vi "GetTileNumberTool.vi"() -> ()   [LabVIEW 2019, in "Initializers.lvlib"]
uses:
  Initializers.lvlib
  <vilib>/Utility/miscctls.llb/LVPositionTypeDef.ctl
panel:
  out "Tilecode":u32=134217750
  in  "Flip":enum16{"None", "LeftRight", "UpDown", "Both"}(ring)
  in  "replace_color 2":fxp<+,3,3>
  in  "color_to_replace 2":fxp<+,3,3>
  out "TileNumber":u32=134217750
  in  "replace_color":fxp<+,3,3>
  in  "color_to_replace":fxp<+,3,3>=2.0
  out "element":picture
  in  "Rotation":enum16{"None", "Right", "Down", "Left"}(ring)
  in  "ReloadFile":bool
  out "Array 2":picture[][](array[picture])=[[bytes[830], bytes[830], bytes[830], bytes[830], bytes[830], bytes[830], bytes[830], bytes[830], bytes[830], bytes[830], bytes[830], bytes[830], bytes[830], bytes[830], bytes[830], bytes[830], bytes[798], bytes[798], bytes[798], bytes[798], bytes[798], bytes[798], bytes[798], bytes[798], bytes[798], bytes[798], bytes[798], bytes[798], bytes[798], bytes[798], bytes[798], bytes[798], bytes[798], bytes[798], bytes[798], bytes[798], bytes[798], bytes[798], bytes[798], bytes[798], bytes[798], bytes[798], bytes[798], bytes[798], bytes[798], bytes[798], bytes[798], bytes[798], bytes[798], bytes[798], bytes[798], bytes[798], bytes[798], bytes[798], bytes[798], bytes[798], bytes[798], bytes[798], bytes[798], bytes[798], bytes[798], bytes[798], bytes[798], bytes[798]], [bytes[830], bytes[830], bytes[830], bytes[830], bytes[830], bytes[830], bytes[830], bytes[830], bytes[830], bytes[830], bytes[830], bytes[830], bytes[830], bytes[830], bytes[830], bytes[830], bytes[798], bytes[798], bytes[798], bytes[798], bytes[798], bytes[798], bytes[798], bytes[798], bytes[798], bytes[798], bytes[798], bytes[798], bytes[798], bytes[798], bytes[798], bytes[798], bytes[798], bytes[798], bytes[798], bytes[798], bytes[798], bytes[798], bytes[798], bytes[798], bytes[798], bytes[798], bytes[798], bytes[798], bytes[798], bytes[798], bytes[798], bytes[798], bytes[798], bytes[798], bytes[798], bytes[798], bytes[798], bytes[798], bytes[798], bytes[798], bytes[798], bytes[798], bytes[798], bytes[798], bytes[798], bytes[798], bytes[798], bytes[798]], [bytes[830], bytes[830], bytes[830], bytes[830], bytes[830], bytes[830], bytes[830], bytes[830], bytes[830], bytes[830], bytes[830], bytes[830], bytes[830], bytes[830], bytes[830], bytes[830], bytes[798], bytes[798], bytes[798], bytes[798], bytes[798], bytes[798], bytes[798], bytes[798], bytes[798], bytes[798], bytes[798], bytes[798], bytes[798], bytes[798], bytes[798], bytes[798], bytes[798], bytes[798], bytes[798], bytes[798], bytes[798], bytes[798], bytes[798], bytes[798], bytes[798], bytes[798], bytes[798], bytes[798], bytes[798], bytes[798], bytes[798], bytes[798], bytes[798], bytes[798], bytes[798], bytes[798], bytes[798], bytes[798], bytes[798], bytes[798], bytes[798], bytes[798], bytes[798], bytes[798], bytes[798], bytes[798], bytes[798], bytes[798]], [bytes[830], bytes[830], bytes[830], bytes[830], bytes[830], bytes[830], bytes[830], bytes[830], bytes[830], bytes[830], bytes[830], bytes[830], bytes[830], bytes[830], bytes[830], bytes[830], bytes[798], bytes[798], bytes[798], bytes[798], bytes[798], bytes[798], bytes[798], bytes[798], bytes[798], bytes[798], bytes[798], bytes[798], bytes[798], bytes[798], bytes[798], bytes[798], bytes[798], bytes[798], bytes[798], bytes[798], bytes[798], bytes[798], bytes[798], bytes[798], bytes[798], bytes[798], bytes[798], bytes[798], bytes[798], bytes[798], bytes[798], bytes[798], bytes[798], bytes[798], bytes[798], bytes[798], bytes[798], bytes[798], bytes[798], bytes[798], bytes[798], bytes[798], bytes[798], bytes[798], bytes[798], bytes[798], bytes[798], bytes[798]], [bytes[830], bytes[830], bytes[830], bytes[830], bytes[830], bytes[830], bytes[830], bytes[830], bytes[830], bytes[830], bytes[830], bytes[830], bytes[830], bytes[830], bytes[830], bytes[830], bytes[798], bytes[798], bytes[798], bytes[798], bytes[798], bytes[798], bytes[798], bytes[798], bytes[798], bytes[798], bytes[798], bytes[798], bytes[798], bytes[798], bytes[798], bytes[798], bytes[798], bytes[798], bytes[798], bytes[798], bytes[798], bytes[798], bytes[798], bytes[798], bytes[798], bytes[798], bytes[798], bytes[798], bytes[798], bytes[798], bytes[798], bytes[798], bytes[798], bytes[798], bytes[798], bytes[798], bytes[798], bytes[798], bytes[798], bytes[798], bytes[798], bytes[798], bytes[798], bytes[798], bytes[798], bytes[798], bytes[798], bytes[798]], [bytes[830], bytes[830], bytes[830], bytes[830], bytes[830], bytes[830], bytes[830], bytes[830], bytes[830], bytes[830], bytes[830], bytes[830], bytes[830], bytes[830], bytes[830], bytes[830], bytes[798], bytes[798], bytes[798], bytes[798], bytes[798], bytes[798], bytes[798], bytes[798], bytes[798], bytes[798], bytes[798], bytes[798], bytes[798], bytes[798], bytes[798], bytes[798], bytes[798], bytes[798], bytes[798], bytes[798], bytes[798], bytes[798], bytes[798], bytes[798], bytes[798], bytes[798], bytes[798], bytes[798], bytes[798], bytes[798], bytes[798], bytes[798], bytes[798], bytes[798], bytes[798], bytes[798], bytes[798], bytes[798], bytes[798], bytes[798], bytes[798], bytes[798], bytes[798], bytes[798], bytes[798], bytes[798], bytes[798], bytes[798]], [bytes[830], bytes[830], bytes[830], bytes[830], bytes[830], bytes[830], bytes[830], bytes[830], bytes[830], bytes[830], bytes[830], bytes[830], bytes[830], bytes[830], bytes[830], bytes[830], bytes[798], bytes[798], bytes[798], bytes[798], bytes[798], bytes[798], bytes[798], bytes[798], bytes[798], bytes[798], bytes[798], bytes[798], bytes[798], bytes[798], bytes[798], bytes[798], bytes[798], bytes[798], bytes[798], bytes[798], bytes[798], bytes[798], bytes[798], bytes[798], bytes[798], bytes[798], bytes[798], bytes[798], bytes[798], bytes[798], bytes[798], bytes[798], bytes[798], bytes[798], bytes[798], bytes[798], bytes[798], bytes[798], bytes[798], bytes[798], bytes[798], bytes[798], bytes[798], bytes[798], bytes[798], bytes[798], bytes[798], bytes[798]], [bytes[830], bytes[830], bytes[830], bytes[830], bytes[830], bytes[830], bytes[830], bytes[830], bytes[830], bytes[830], bytes[830], bytes[830], bytes[830], bytes[830], bytes[830], bytes[830], bytes[798], bytes[798], bytes[798], bytes[798], bytes[798], bytes[798], bytes[798], bytes[798], bytes[798], bytes[798], bytes[798], bytes[798], bytes[798], bytes[798], bytes[798], bytes[798], bytes[798], bytes[798], bytes[798], bytes[798], bytes[798], bytes[798], bytes[798], bytes[798], bytes[798], bytes[798], bytes[798], bytes[798], bytes[798], bytes[798], bytes[798], bytes[798], bytes[798], bytes[798], bytes[798], bytes[798], bytes[798], bytes[798], bytes[798], bytes[798], bytes[798], bytes[798], bytes[798], bytes[798], bytes[798], bytes[798], bytes[798], bytes[798]], [bytes[830], bytes[830], bytes[830], bytes[830], bytes[830], bytes[830], bytes[830], bytes[830], bytes[830], bytes[830], bytes[830], bytes[830], bytes[830], bytes[830], bytes[830], bytes[830], bytes[798], bytes[798], bytes[798], bytes[798], bytes[798], bytes[798], bytes[798], bytes[798], bytes[798], bytes[798], bytes[798], bytes[798], bytes[798], bytes[798], bytes[798], bytes[798], bytes[798], bytes[798], bytes[798], bytes[798], bytes[798], bytes[798], bytes[798], bytes[798], bytes[798], bytes[798], bytes[798], bytes[798], bytes[798], bytes[798], bytes[798], bytes[798], bytes[798], bytes[798], bytes[798], bytes[798], bytes[798], bytes[798], bytes[798], bytes[798], bytes[798], bytes[798], bytes[798], bytes[798], bytes[798], bytes[798], bytes[798], bytes[798]], [bytes[830], bytes[830], bytes[830], bytes[830], bytes[830], bytes[830], bytes[830], bytes[830], bytes[830], bytes[830], bytes[830], bytes[830], bytes[830], bytes[830], bytes[830], bytes[830], bytes[798], bytes[798], bytes[798], bytes[798], bytes[798], bytes[798], bytes[798], bytes[798], bytes[798], bytes[798], bytes[798], bytes[798], bytes[798], bytes[798], bytes[798], bytes[798], bytes[798], bytes[798], bytes[798], bytes[798], bytes[798], bytes[798], bytes[798], bytes[798], bytes[798], bytes[798], bytes[798], bytes[798], bytes[798], bytes[798], bytes[798], bytes[798], bytes[798], bytes[798], bytes[798], bytes[798], bytes[798], bytes[798], bytes[798], bytes[798], bytes[798], bytes[798], bytes[798], bytes[798], bytes[798], bytes[798], bytes[798], bytes[798]], [bytes[830], bytes[830], bytes[830], bytes[830], bytes[830], bytes[830], bytes[830], bytes[830], bytes[830], bytes[830], bytes[830], bytes[830], bytes[830], bytes[830], bytes[830], bytes[830], bytes[798], bytes[798], bytes[798], bytes[798], bytes[798], bytes[798], bytes[798], bytes[798], bytes[798], bytes[798], bytes[798], bytes[798], bytes[798], bytes[798], bytes[798], bytes[798], bytes[798], bytes[798], bytes[798], bytes[798], bytes[798], bytes[798], bytes[798], bytes[798], bytes[798], bytes[798], bytes[798], bytes[798], bytes[798], bytes[798], bytes[798], bytes[798], bytes[798], bytes[798], bytes[798], bytes[798], bytes[798], bytes[798], bytes[798], bytes[798], bytes[798], bytes[798], bytes[798], bytes[798], bytes[798], bytes[798], bytes[798], bytes[798]], [bytes[830], bytes[830], bytes[830], bytes[830], bytes[830], bytes[830], bytes[830], bytes[830], bytes[830], bytes[830], bytes[830], bytes[830], bytes[830], bytes[830], bytes[830], bytes[830], bytes[798], bytes[798], bytes[798], bytes[798], bytes[798], bytes[798], bytes[798], bytes[798], bytes[798], bytes[798], bytes[798], bytes[798], bytes[798], bytes[798], bytes[798], bytes[798], bytes[798], bytes[798], bytes[798], bytes[798], bytes[798], bytes[798], bytes[798], bytes[798], bytes[798], bytes[798], bytes[798], bytes[798], bytes[798], bytes[798], bytes[798], bytes[798], bytes[798], bytes[798], bytes[798], bytes[798], bytes[798], bytes[798], bytes[798], bytes[798], bytes[798], bytes[798], bytes[798], bytes[798], bytes[798], bytes[798], bytes[798], bytes[798]], [bytes[830], bytes[830], bytes[830], bytes[830], bytes[830], bytes[830], bytes[830], bytes[830], bytes[830], bytes[830], bytes[830], bytes[830], bytes[830], bytes[830], bytes[830], bytes[830], bytes[798], bytes[798], bytes[798], bytes[798], bytes[798], bytes[798], bytes[798], bytes[798], bytes[798], bytes[798], bytes[798], bytes[798], bytes[798], bytes[798], bytes[798], bytes[798], bytes[798], bytes[798], bytes[798], bytes[798], bytes[798], bytes[798], bytes[798], bytes[798], bytes[798], bytes[798], bytes[798], bytes[798], bytes[798], bytes[798], bytes[798], bytes[798], bytes[798], bytes[798], bytes[798], bytes[798], bytes[798], bytes[798], bytes[798], bytes[798], bytes[798], bytes[798], bytes[798], bytes[798], bytes[798], bytes[798], bytes[798], bytes[798]], [bytes[830], bytes[830], bytes[830], bytes[830], bytes[830], bytes[830], bytes[830], bytes[830], bytes[830], bytes[830], bytes[830], bytes[830], bytes[830], bytes[830], bytes[830], bytes[830], bytes[798], bytes[798], bytes[798], bytes[798], bytes[798], bytes[798], bytes[798], bytes[798], bytes[798], bytes[798], bytes[798], bytes[798], bytes[798], bytes[798], bytes[798], bytes[798], bytes[798], bytes[798], bytes[798], bytes[798], bytes[798], bytes[798], bytes[798], bytes[798], bytes[798], bytes[798], bytes[798], bytes[798], bytes[798], bytes[798], bytes[798], bytes[798], bytes[798], bytes[798], bytes[798], bytes[798], bytes[798], bytes[798], bytes[798], bytes[798], bytes[798], bytes[798], bytes[798], bytes[798], bytes[798], bytes[798], bytes[798], bytes[798]], [bytes[830], bytes[830], bytes[830], bytes[830], bytes[830], bytes[830], bytes[830], bytes[830], bytes[830], bytes[830], bytes[830], bytes[830], bytes[830], bytes[830], bytes[830], bytes[830], bytes[798], bytes[798], bytes[798], bytes[798], bytes[798], bytes[798], bytes[798], bytes[798], bytes[798], bytes[798], bytes[798], bytes[798], bytes[798], bytes[798], bytes[798], bytes[798], bytes[798], bytes[798], bytes[798], bytes[798], bytes[798], bytes[798], bytes[798], bytes[798], bytes[798], bytes[798], bytes[798], bytes[798], bytes[798], bytes[798], bytes[798], bytes[798], bytes[798], bytes[798], bytes[798], bytes[798], bytes[798], bytes[798], bytes[798], bytes[798], bytes[798], bytes[798], bytes[798], bytes[798], bytes[798], bytes[798], bytes[798], bytes[798]], [bytes[830], bytes[830], bytes[830], bytes[830], bytes[830], bytes[830], bytes[830], bytes[830], bytes[830], bytes[830], bytes[830], bytes[830], bytes[830], bytes[830], bytes[830], bytes[830], bytes[798], bytes[798], bytes[798], bytes[798], bytes[798], bytes[798], bytes[798], bytes[798], bytes[798], bytes[798], bytes[798], bytes[798], bytes[798], bytes[798], bytes[798], bytes[798], bytes[798], bytes[798], bytes[798], bytes[798], bytes[798], bytes[798], bytes[798], bytes[798], bytes[798], bytes[798], bytes[798], bytes[798], bytes[798], bytes[798], bytes[798], bytes[798], bytes[798], bytes[798], bytes[798], bytes[798], bytes[798], bytes[798], bytes[798], bytes[798], bytes[798], bytes[798], bytes[798], bytes[798], bytes[798], bytes[798], bytes[798], bytes[798]]]
  in  "path to PNG file":path=path "C:/Users/FreshBob/Dropbox/VIs/myRIO_GameConsole/Data/Tilesets/UnifiedTileset.png"
  in  "stop":bool
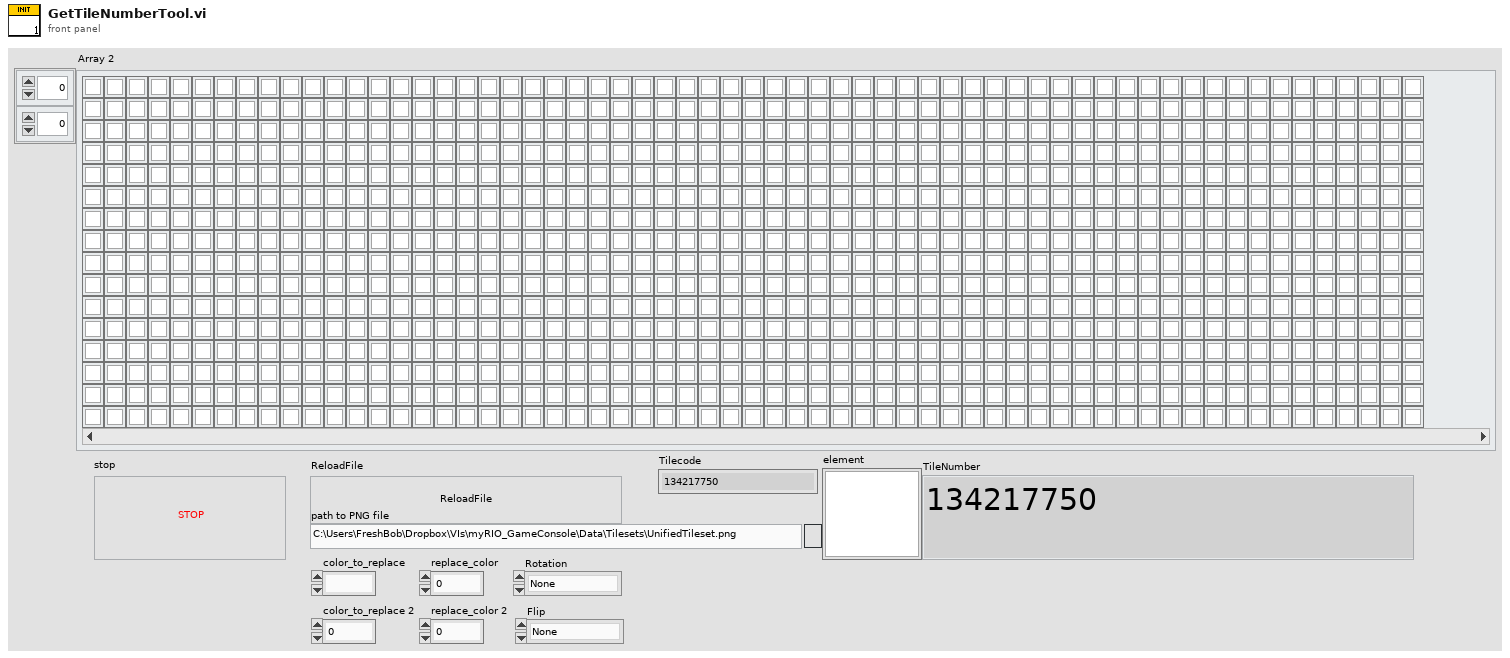
[diagram p1: front panel]
types:
  T1 = typedef "LVPositionTypeDef.ctl" = cluster{"Left":i32, "Top":i32}
  T2 = cluster{"left":i16, "top":i16, "right":i16, "bottom":i16}
  T3 = typedef "LVPoint32TypeDef.ctl" = cluster{"Horizontal":i32, "Vertical":i32}
  T4 = typedef "LVBoundsTypeDef.ctl" = cluster{"Width":u32, "Height":u32}
  T5 = typedef "imagedata.ctl" = cluster{"image type":i32, "image depth":i32, "image":u8[], "mask":u8[], "colors":u32[], "Rectangle":cluster{"left":i16, "top":i16, "right":i16, "bottom":i16}}
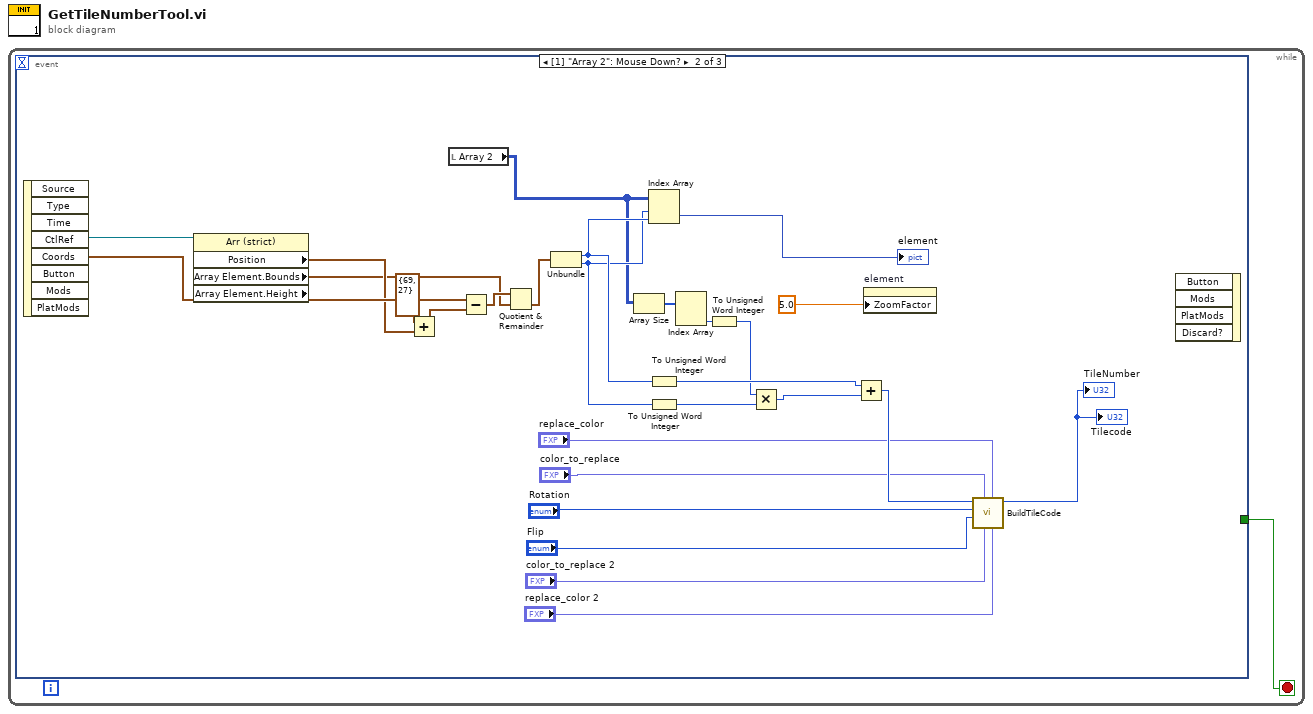
[diagram p0: block diagram]
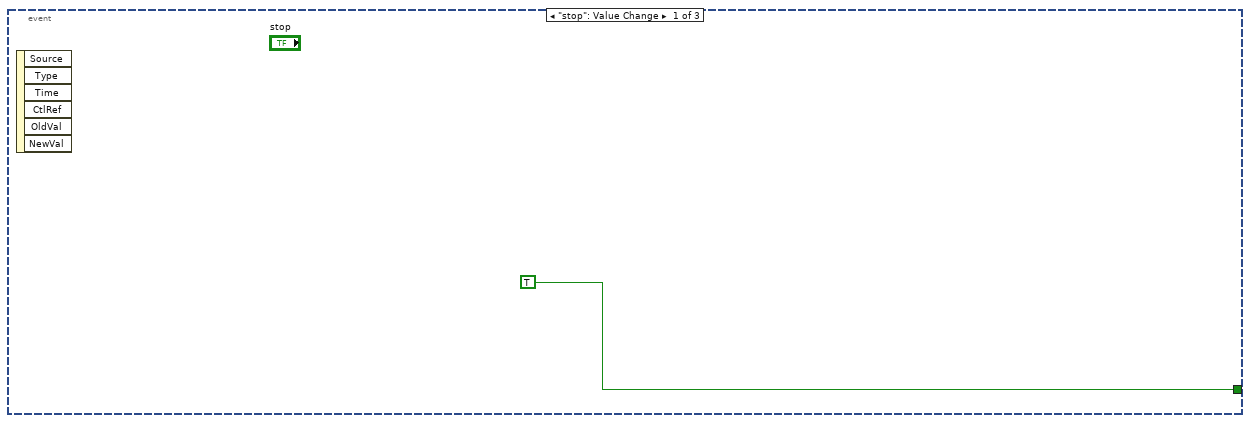
[diagram p2: hidden frame]
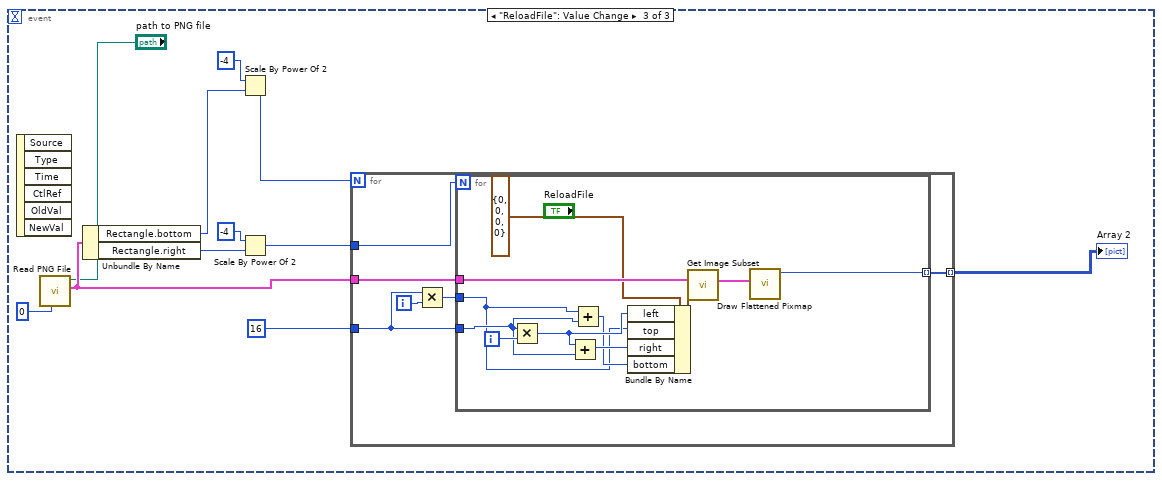
[diagram p3: hidden frame]
diagram:
  n1 = while {
    stop <- w1 stop-if-true
    n2 = event shown="[1] \"Array 2\": Mouse Down?" {
      selector: _ -> [_ _ _]
      dyn-events: _ -> [_ _ _]
      timeout: _ -> [_ _ _]
      tunnel: [TRUE _ _] -> w1
      event "stop": Value Change {
        n3 = event-data() -> ()  [unwired: 1 in, 6 out]
      }
      event "Array 2": Mouse Down? {
        n4 = event-data() -> ("CtlRef"=w29:refnum<vi>, "Coords"=w28:T3)  [unwired: 1 in, 6 out]
        n5 = property class="Arr (strict)" props=["Position", "Array Element", "Bounds", "Array Element", "Height"](reference=w29) -> ("Position"=w27:T1, "Array Element.Bounds"=w25:T4)  [unwired: 1 in, 3 out]
        n6 = Add(x=T1 {"Left"=69, "Top"=27}, y=w27) -> (x+y=w24:T1)
        n7 = local read "Array 2"() -> (w17:picture[][])
        n8 = Subtract(x=w28, y=w24) -> (x-y=w26:T3)
        n9 = Quotient & Remainder(x=w26, y=w25) -> (floor(x/y)=w22:T4)  [unwired: 1 out]
        n10 = Unbundle(w22) -> ("Width"=w19:u32, "Height"=w18:u32)
        n11 = Array Size(array=w17) -> (size(s)=w16:i32[])
        n12 = Index Array(array=w17, index (row)=w18, index (col)=w19) -> (element=→"element":picture)
        n13 = To Unsigned Word Integer(number=w19) -> (unsigned 16bit integer=w12:u16)
        n14 = To Unsigned Word Integer(number=w18) -> (unsigned 16bit integer=w15:u16)
        n15 = Index Array(array=w16) -> (element #2=w14:i32)  [unwired: 2 in, 1 out]
        n16 = To Unsigned Word Integer(number=w14) -> (unsigned 16bit integer=w11:u16)
        n17 = Multiply(x=w11, y=w15) -> (x*y=w13:u16)
        n18 = Add(x=w12, y=w13) -> (x+y=w9:u16)
        n19 = property on="element" class="Pict"("ZoomFactor"=sgl 5.0 ("Zoom Factor")) -> ()  [unwired: 2 in, 2 out]
        n20 = call "BuildTileCode.vi"("replacecolor 2"="replace_color 2", "replacecolor"="replace_color", "color_to_replace 2"="color_to_replace 2", "color_to_replace"="color_to_replace", "Flip"="Flip", "Rotation"="Rotation", "Tilenumber"=w9) -> ("Tilecode"=→"TileNumber" →"Tilecode":u32)  [unwired: 4 in]
        n21 = event-data() -> ()  [unwired: 5 in, 1 out]
      }
      event "ReloadFile": Value Change {
        n22 = event-data() -> ()  [unwired: 1 in, 6 out]
        n23 = call <vilib>:"Read PNG File.vi"("Transparency Thresh"=u8 0, "path to PNG file"="path to PNG file") -> ("image data"=w40:T5)  [unwired: 7 in, 2 out]
        n24 = Unbundle By Name(w40) -> ("Rectangle.bottom"=w36:i16, "Rectangle.right"=w33:i16)
        n25 = Scale By Power Of 2(n=i16 -4, x=w36) -> (x*2^n=w31:i16)
        n26 = Scale By Power Of 2(n=i16 -4, x=w33) -> (x*2^n=w32:i16)
        n27 = for {
          N: w31 -> [_]
          tunnel: w40 -> [w46]
          tunnel: 16 ("length") -> [w44]
          tunnel: w32 -> [w42]
          tunnel: [w41] -> w30 mode=indexing
          i -> [w45]
          n28 = Multiply(x=w44, y=w45) -> (x*y=w43:i32)
          n29 = for {
            N: w42 -> [_]
            tunnel: w46 -> [w57]
            tunnel: w44 -> [w48]
            tunnel: w43 -> [w47]
            tunnel: [w51] -> w41 mode=indexing
            i -> [w54]
            n30 = Multiply(x=w48, y=w54) -> (x*y=w53:i32)
            n31 = Add(x=w53, y=w48) -> (x+y=w50:i32)
            n32 = Add(x=w47, y=w48) -> (x+y=w49:i32)
            n33 = Bundle By Name(cluster=T2 {"left"=0, "top"=0, "right"=0, "bottom"=0} ("subset rect"), "left"=w53, "top"=w47, "right"=w50, "bottom"=w49) -> (w55:T2)
            n34 = call <vilib>:"Get Image Subset.vi"("subset rect"=w55, "image data"=w57) -> ("image subset"=w52:T5)  [unwired: 4 in, 1 out]
            n35 = call <vilib>:"Draw Flattened Pixmap.vi"("image data"=w52) -> ("new picture"=w51:picture)  [unwired: 8 in]
          }
        }
        "Array 2" <- w30
      }
    }
  }
